vi "ProcessMatlabEvents.vi"(8 "Event Wait timeout":i32=10, 11 "ExperimentID":string) -> ()   [LabVIEW 2017]
uses:
  Types/MatlabDataBundle.ctl
  Types/MatlabDataType.ctl
  Types/MatlabBindingDirectionEnum.ctl
  Types/MethodInvokeInfo.ctl
panel:
  out "Checking changes on control":string
  out "Matlab Param Data":T1[](array[typedef])
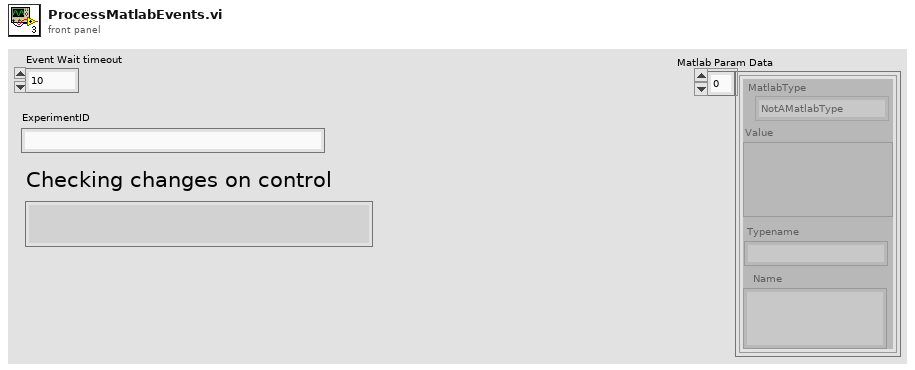
[diagram p1: front panel]
types:
  T1 = typedef "MatlabDataBundle.ctl" = cluster{"MatlabType":T2, "Value":variant, "Name":string, "Typename":string}
  T2 = typedef "MatlabDataType.ctl" = enum16{"NotAMatlabType", "Real", "Complex", "String", "Boolean"}
  T3 = typedef "MatlabBindingDirectionEnum.ctl" = enum16{"BiDirectional", "FromMatlab", "ToMatlab"}
  T4 = typedef "MethodInvokeInfo.ctl" = cluster{"Method Name":string, "Arguments":variant}
  T5 = typedef "ControlValueChangeEventBindingType.ctl" = cluster{"Control":refnum<vi>, "Event Register":refnum<event-registration>, "AllowVariantValues":bool, "Direction":T3}
  T6 = typedef "MatlabEventStruct.ctl" = cluster{"Name":string, "DataIndex":dbl, "Category":string, "Matlab Param Data":T1[]}
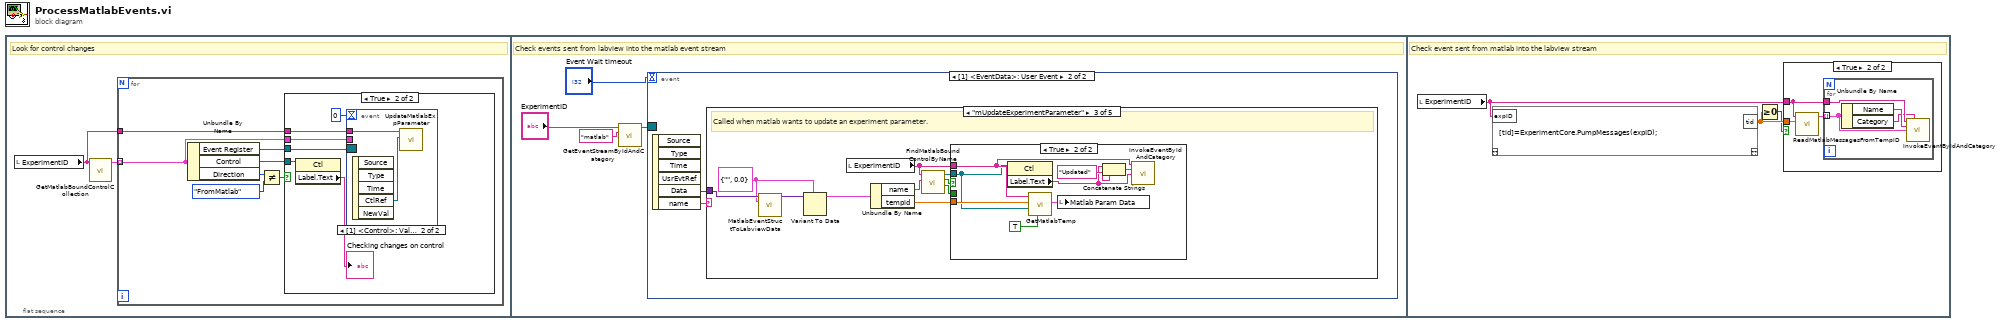
[diagram p0: block diagram]
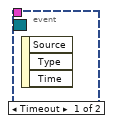
[diagram p3: hidden frame]
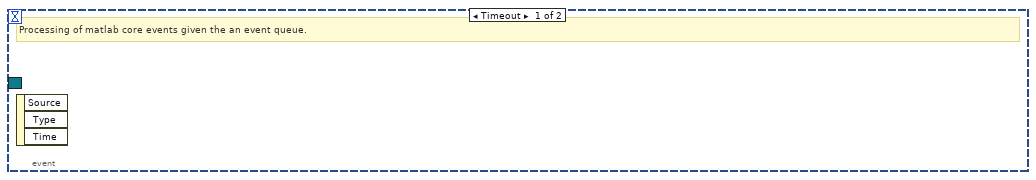
[diagram p4: hidden frame]
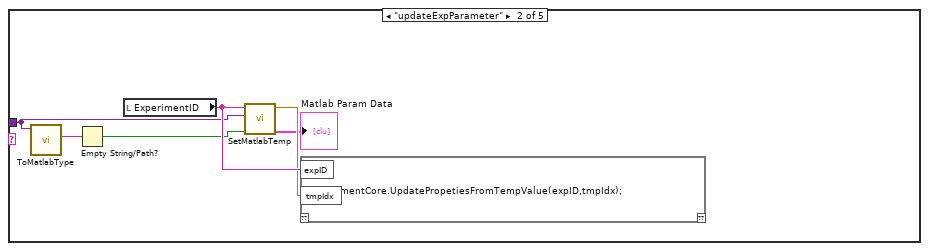
[diagram p6: hidden frame]
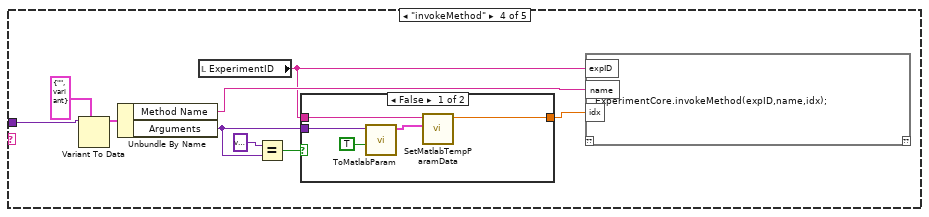
[diagram p8: hidden frame]
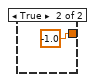
[diagram p9: hidden frame]
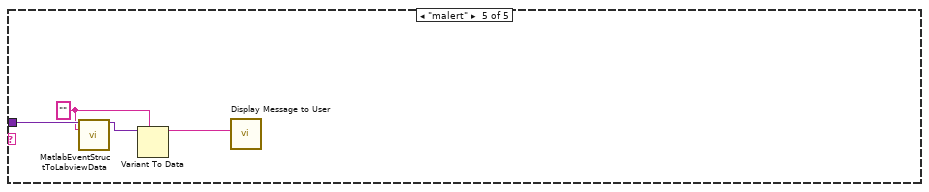
[diagram p10: hidden frame]
diagram:
  n1 = flat-sequence {
    frame #0 {
      # "Look for control changes"
      n2 = local read "ExperimentID"() -> (w1:string)
      n3 = call "GetMatlabBoundControlCollection.vi"("ExpID"=w1) -> ("Bound Controls"=w2:T5[])  [unwired: 10 in]
      n4 = for {
        tunnel: w2 -> [w7] mode=indexing
        tunnel: w1 -> [w8]
        n5 = Unbundle By Name(w7) -> ("Event Register"=w9:refnum<event-registration>, "Control"=w6:refnum<vi>, "Direction"=w4:T3)
        n6 = Not Equal?(x=w4, y=MatlabBindingDirectionEnum."FromMatlab" ("Direction")) -> (x != y?=w3:bool)
        n7 = case shown="True" w3 {
          tunnel: w9 -> [_ w15]
          tunnel: w8 -> [_ w14]
          tunnel: w7 -> [_ w13]
          tunnel: w6 -> [_ w11]
          frame False {
          }
          frame True {
            n8 = property class="Ctl"(reference=w11) -> ("Label.Text"=→"Checking changes on control":string)  [unwired: 1 in, 2 out]
            n9 = event shown="[1] <Control>: Value Change" {
              selector: w15 -> [_ _]
              dyn-events: _ -> [_ _]
              timeout: 0 -> [_ _]
              tunnel: w14 -> [_ w17]
              tunnel: w13 -> [_ _]
              event Timeout {
                n10 = event-data() -> ()  [unwired: 1 in, 3 out]
              }
              event Value Change {
                n11 = event-data() -> ("CtlRef"=w16:refnum<vi>)  [unwired: 1 in, 4 out]
                n12 = call "UpdateMatlabExpParameter.vi"("Parameter(s)"=w16, "ExpID"=w17) -> ()  [unwired: 9 in, 1 out]
              }
            }
          }
        }
      }
    }
    frame #1 {
      # "Check events sent from labview into the matlab event stream"
      n13 = call "GetEventStreamByIdAndCategory.vi"("Category"="matlab", "ID"="ExperimentID") -> ("Event Registration Refnum out"=w19:refnum<event-registration>)  [unwired: 7 in, 2 out]
      n14 = event shown="[1] <EventData>: User Event" {
        selector: w19 -> [_ _]
        dyn-events: _ -> [_ _]
        timeout: "Event Wait timeout" -> [_ _]
        event Timeout {
          # "Processing of matlab core events given the an event queue."
          n15 = event-data() -> ()  [unwired: 1 in, 3 out]
        }
        event User Event {
          n16 = event-data() -> ("Data"=w22:variant, "name"=w23:string)  [unwired: 1 in, 4 out]
          n17 = case shown="\"mUpdateExperimentParameter\"" w23 {
            tunnel: w22 -> [_ w27 w38 w55 w66]
            frame "False", Default {
            }
            frame "updateExpParameter" {
              n18 = call "ToMatlabType.vi"("Value"=w27) -> ("Name"=w26:string)  [unwired: 7 in, 3 out]
              n19 = Empty String/Path?(string/path=w26) -> (empty?=w25:bool)
              n20 = local read "ExperimentID"() -> (w29:string)
              n21 = call "SetMatlabTemp.vi"("IgnoreContainerName"=w25, "Variant"=w27, "ExpID"=w29) -> ("Matlab Param Data"=→"Matlab Param Data":T1[], "index out"=w28:dbl)  [unwired: 7 in]
              n22 = script code="ExperimentCore.UpdatePropetiesFromTempValue(expID,tmpIdx);"("expID"=w29, "tmpIdx"=w28) -> ()  [unwired: 1 in, 1 out]
            }
            frame "mUpdateExperimentParameter" {
              w37 = cluster{"name":string, "tempid":dbl} {"name"="", "tempid"=0.0}
              # "Called when matlab wants to update an experiment parameter."
              n23 = call "MatlabEventStructToLabviewData.vi"("Event Variant"=w38, "Value to update (or object type)"=w37) -> ("Value"=w39:variant)  [unwired: 11 in, 2 out]
              n24 = Variant To Data(type=w37, Variant=w39) -> (data=w36:cluster{"name":string, "tempid":dbl})  [unwired: 1 in, 1 out]
              n25 = local read "ExperimentID"() -> (w31:string)
              n26 = Unbundle By Name(w36) -> ("name"=w35:string, "tempid"=w33:dbl)
              n27 = call "FindMatlabBoundControlByName.vi"("name"=w35, "ExperimentID"=w31) -> ("AllowVariantValues"=w30:bool, "Boolean"=w34:bool, "Control out"=w32:refnum<vi>)  [unwired: 7 in]
              n28 = case shown="True" w34 {
                tunnel: w33 -> [_ w47]
                tunnel: w32 -> [_ w40]
                tunnel: w31 -> [_ w44]
                tunnel: w30 -> [_ _]
                frame False {
                }
                frame True {
                  n29 = property class="Ctl"(reference=w40) -> ("Label.Text"=w42:string)  [unwired: 1 in, 2 out]
                  n30 = call "GetMatlabTemp.vi"("IgnoreContainerName"=TRUE, "Value To Update (or type)"=w40, "index in"=w47, "ExpID"=w44) -> ("Matlab param data"=w45:T1[])  [unwired: 5 in, 2 out]
                  n31 = local write "Matlab Param Data"(w45) -> ()
                  n32 = Concatenate Strings(w42, "Updated" ("eventName")) -> (w41:string)
                  n33 = call "InvokeEventByIdAndCategory.vi"("ID"=w44, "eventName"=w41, "Data"=w42) -> ()  [unwired: 12 in, 1 out]
                }
              }
            }
            frame "invokeMethod" {
              n34 = Variant To Data(type=T4 {"Method Name"="", "Arguments"=variant} ("Method Invoke Info"), Variant=w55) -> (data=w54:T4)  [unwired: 1 in, 1 out]
              n35 = Unbundle By Name(w54) -> ("Method Name"=w49:string, "Arguments"=w50:variant)
              n36 = local read "ExperimentID"() -> (w48:string)
              n37 = Equal?(x=variant, y=w50) -> (x = y?=w51:bool)
              n38 = case shown="False" w51 {
                tunnel: [w59 -1.0] -> w52
                tunnel: w50 -> [w60 _]
                tunnel: w48 -> [w57 _]
                frame False {
                  n39 = call "ToMatlabParam.vi"("IgnoreContainerName"=TRUE, "Value"=w60) -> ("Matlab Param Data"=w61:T1[])  [unwired: 9 in]
                  n40 = call "SetMatlabTempParamData.vi"("Matlab param data"=w61, "ExperimentID"=w57) -> ("index out"=w59:dbl)  [unwired: 9 in]
                }
                frame True {
                }
              }
              n41 = script code="ExperimentCore.invokeMethod(expID,name,idx);"("expID"=w48, "name"=w49, "idx"=w52) -> ()  [unwired: 1 in, 1 out]
            }
            frame "malert" {
              w63 = ""
              n42 = call "MatlabEventStructToLabviewData.vi"("Event Variant"=w66, "Value to update (or object type)"=w63) -> ("Value"=w65:variant)  [unwired: 11 in, 2 out]
              n43 = Variant To Data(type=w63, Variant=w65) -> (data=w64:string)  [unwired: 1 in, 1 out]
              n44 = call "Display Message to User"("Message"=w64) -> ()  [unwired: 9 in, 2 out]
            }
          }
        }
      }
    }
    frame #2 {
      # "Check event sent from matlab into the labview stream"
      n45 = local read "ExperimentID"() -> (w69:string)
      n46 = script code="[tid]=ExperimentCore.PumpMessages(expID);"("expID"=w69) -> ("tid"=w68:dbl)  [unwired: 1 in, 1 out]
      n47 = Greater Or Equal To 0?(x=w68) -> (x >= 0?=w67:bool)
      n48 = case shown="True" w67 {
        tunnel: w68 -> [_ w72]
        tunnel: w69 -> [_ w70]
        frame False {
        }
        frame True {
          n49 = call "ReadMatlabMessagesFromTempID.vi"("Numeric"=w72, "ExperimentID"=w70) -> ("Read messages"=w71:T6[])  [unwired: 9 in]
          n50 = for {
            tunnel: w71 -> [w74] mode=indexing
            tunnel: w70 -> [w76]
            n51 = Unbundle By Name(w74) -> ("Name"=w75:string, "Category"=w73:string)
            n52 = call "InvokeEventByIdAndCategory.vi"("ID"=w76, "Category"=w73, "eventName"=w75, "Data"=w74) -> ()  [unwired: 11 in, 1 out]
          }
        }
      }
    }
  }
